vi "Get Drive Type.vi"(7 "error in (no error)":errorcluster, 10 "Root Path name (C:\\)":string="c:\\") -> (0 "error out":errorcluster, 2 "Drive Type":T1(ring), 3 "Dup Root Path name (C:\\)":string="c:\\")   [LabVIEW 2012, in "API.lvlib"]
doc: "Retrieves the type of the requested drive.\nMay be one of the following....\n0:Unkown\n1:No Root\n2:Removable\n3:Fixed\n4:Remote\n5:CD Rom\n6:Ramdisk"
uses:
  API.lvlib
  kernel32.dll
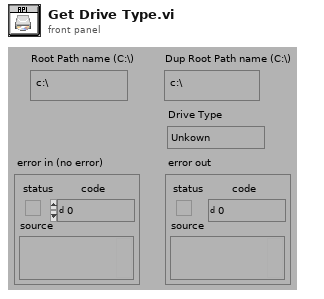
[diagram p1: front panel]
types:
  T1 = enum16{"Unkown", "No Root", "Removable", "Fixed", "Remote", "CD Rom", "Ramdisk"}
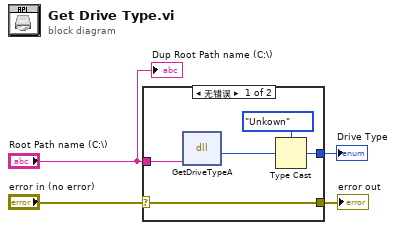
[diagram p0: block diagram]
diagram:
  n1 = case shown="无错误" "error in (no error)" {
    selector: "error in (no error)" -> [w6 w10]
    tunnel: "Root Path name (C:\\)" -> [w9 _]
    tunnel: [w7 _] -> w1
    tunnel: [w6 w10] -> w2
    frame No Error {
      n2 = dll-call lib="kernel32.dll" fn="GetDriveTypeA" ("GetDrive Type")("lpRootPathName"=w9) -> (w8:u16)  [unwired: 4 in, 2 out]
      n3 = Type Cast(type=T1."Unkown" ("Drive Type"), x=w8) -> (*(type *) &x=w7:T1)
    }
    frame Error {
    }
  }
  "Drive Type" <- w1
  "error out" <- w2
  "Dup Root Path name (C:\\)" <- "Root Path name (C:\\)"
